vi "FindFaces.vi"(7 "File Path":path, 8 "error in":errorcluster, 9 "Face Cascade Path":path, 11 "Image In":T1) -> (0 "error out":errorcluster, 3 "Array":T1[](array[typedef]))   [LabVIEW 2019]
uses:
  <vilib>/vision/Image Controls.llb/IMAQ Image.ctl
  <vilib>/vision/NI_Vision_Development_Module.lvlib
panel:
  in  "index":i32
  out "Image 2":T1(plugin-control)
  out "size(s)":i32
  out "Image":T1(plugin-control)
  out "Faces":T2[](array[typedef]) {"Rotation" format="%.2f"; "Left" scale=0.0..1024.0; "Right" scale=0.0..1024.0}
  in  "Eyes Cascade Path":path
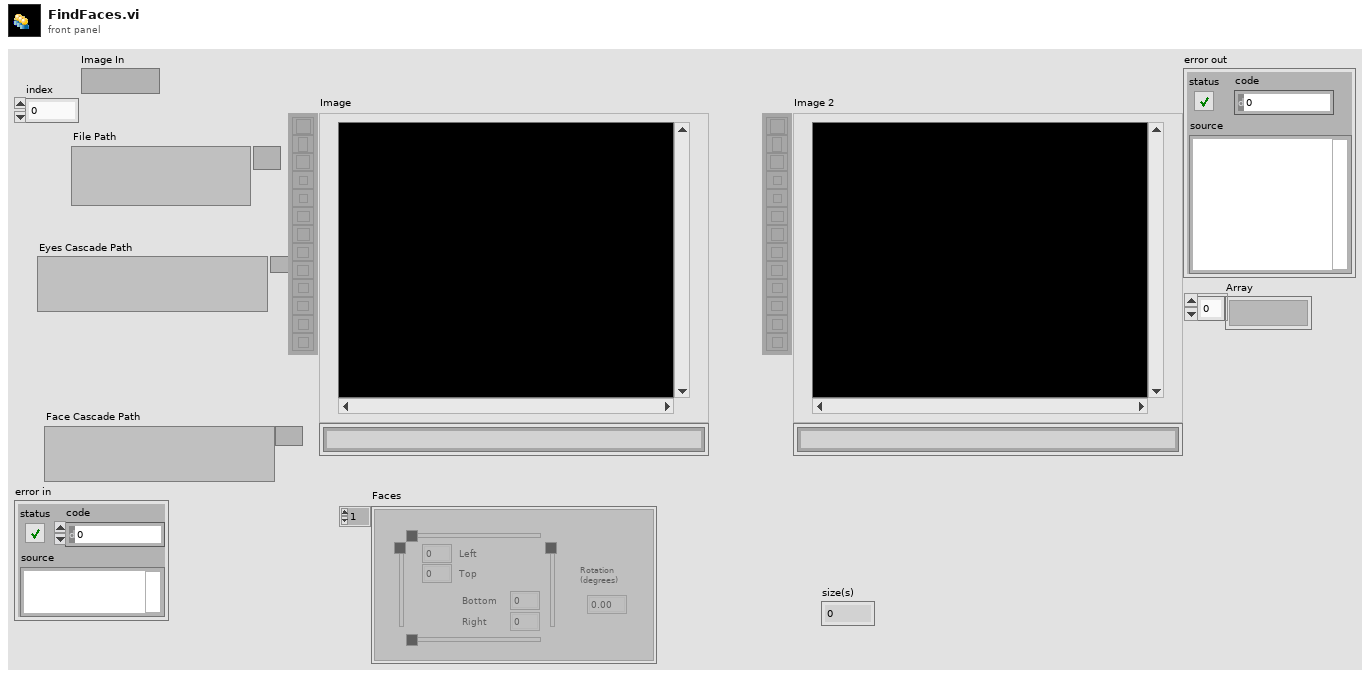
[diagram p1: front panel]
types:
  T1 = typedef "IMAQ Image.ctl" = refnum<image>
  T2 = typedef "IMAQ Rectangle" = cluster{"Left":i32, "Top":i32, "Right":i32, "Bottom":i32, "Rotation":dbl}
  T3 = typedef "Image Type" = u32
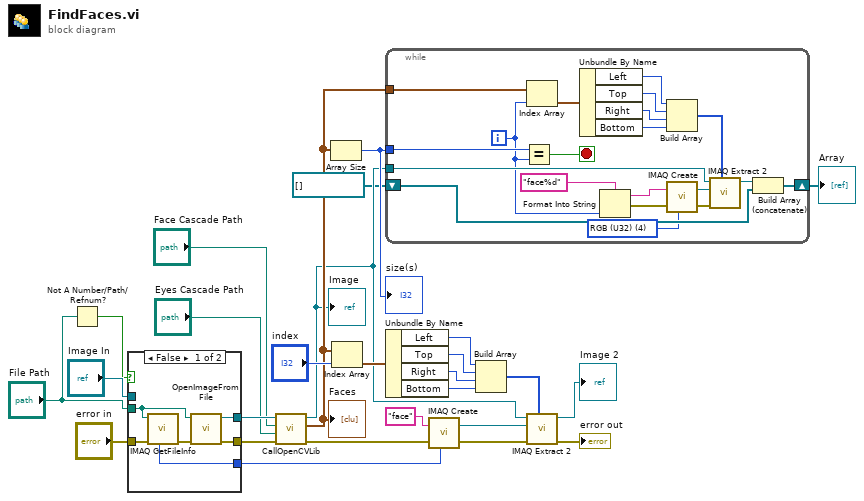
[diagram p0: block diagram]
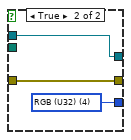
[diagram p2: hidden frame]
diagram:
  n1 = Not A Number/Path/Refnum?(number/path/refnum="File Path") -> (NaN/Path/Refnum?=w21:bool)
  n2 = case shown="False" w21 {
    tunnel: "File Path" -> [w31 _]
    tunnel: [w33 w35] -> w27
    tunnel: [w32 w34] -> w26
    tunnel: [w30 w36] -> w23
    tunnel: "Image In" -> [_ w35]
    tunnel: "error in" -> [w29 w34]
    frame False {
      n3 = call "IMAQ GetFileInfo"("error in (no error)"=w29, "File Path"=w31) -> ("error out"=w28:errorcluster, "Image Type"=w30:T3)  [unwired: 8 out]
      n4 = call "OpenImageFromFile.vi"("error in (no error)"=w28, "File Path"=w31) -> ("error out"=w32:errorcluster, "Image"=w33:T1)  [unwired: 8 in]
    }
    frame True {
      w36 = T3 4 items=["Grayscale (U8)", "Grayscale (I16)", "Grayscale (SGL)", "Complex (CSG)", "RGB (U32)", "HSL (U32)", "RGB (U64)", "Grayscale (U16)"] ("Image Type")
    }
  }
  n5 = call "CallOpenCVLib.vi"("error in (no error)"=w26, "Eyes Cascade Path"="Eyes Cascade Path", "Face Cascade Path"="Face Cascade Path", "Image Src"=w27) -> ("error out"=w17:errorcluster, "Faces"=w5:T2[], "Image Dst Out"=w3:T1)  [unwired: 4 in, 1 out]
  "Faces" <- w5
  "Image" <- w3
  n6 = Array Size(array=w5) -> (size(s)=w4:i32)
  "size(s)" <- w4
  n7 = Index Array(array=w5, index="index") -> (element=w10:T2)
  n8 = while {
    tunnel: w5 -> [w54]
    tunnel: w4 -> [w55]
    tunnel: w3 -> [w48]
    shift-right: [w39] -> w1
    shift-left: T1[] [] -> [w38]
    i -> [w41]
    stop <- w56 stop-if-true
    w37 = T3 4 items=["Grayscale (U8)", "Grayscale (I16)", "Grayscale (SGL)", "Complex (CSG)", "RGB (U32)", "HSL (U32)", "RGB (U64)", "Grayscale (U16)"] ("Image Type")
    n9 = Equal?(x=w55, y=w41) -> (x = y?=w56:bool)
    n10 = Index Array(array=w54, index=w41) -> (element=w49:T2)
    n11 = Unbundle By Name(w49) -> ("Left"=w53:i32, "Top"=w52:i32, "Right"=w51:i32, "Bottom"=w50:i32)
    n12 = Format Into String(format string="face%d" ("Image Name"), w41) -> (resulting string=w43:string, error out=w44:errorcluster)  [unwired: 2 in]
    n13 = Build Array(w53, w52, w51, w50) -> (w47:i32[])
    n14 = call "IMAQ Create"("Image Name"=w43, "Image Type"=w37, "error in (no error)"=w44) -> ("New Image"=w46:T1, "error out"=w45:errorcluster)  [unwired: 2 in]
    n15 = call "IMAQ Extract 2"("Optional Rectangle"=w47, "error in (no error)"=w45, "Image Dst"=w46, "Image Src"=w48) -> ("Image Dst Out"=w40:T1)  [unwired: 6 in, 1 out]
    n16 = Build Array (concatenate)(w40, w38) -> (w39:T1[])
  }
  "Array" <- w1
  n17 = Unbundle By Name(w10) -> ("Left"=w11:i32, "Top"=w12:i32, "Right"=w13:i32, "Bottom"=w14:i32)
  n18 = call "IMAQ Create"("Image Name"="face", "Image Type"=w23, "error in (no error)"=w17) -> ("New Image"=w6:T1, "error out"=w18:errorcluster)  [unwired: 2 in]
  n19 = Build Array(w11, w12, w13, w14) -> (w15:i32[])
  n20 = call "IMAQ Extract 2"("Optional Rectangle"=w15, "error in (no error)"=w18, "Image Dst"=w6, "Image Src"=w3) -> ("error out"=→"error out":errorcluster, "Image Dst Out"=→"Image 2":T1)  [unwired: 6 in]
